vi "Get LV Timestamp Format String.vi"() -> (0 "timestamp string format":string="%Y-%m-%dT%H:%M:%S%3u%z")   [LabVIEW 2021, in "Logging.lvlib"]
doc: "Get the nearest-compliant format string for ISO 8601 that LabVIEW supports. After formatting a timestamp, use \"Fix LV Timestamp String.vi\" to make the formatted timestamp compliant with ISO 8601."
uses:
  Logging.lvlib
panel:
  out "Now":string
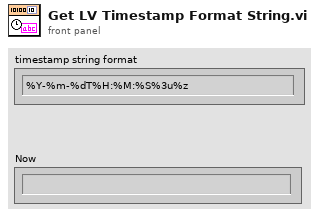
[diagram p1: front panel]
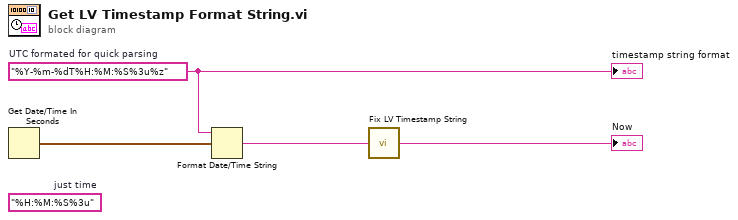
[diagram p0: block diagram]
diagram:
  (unwired) "%H:%M:%S%3u"  # just time
  w3 = "%Y-%m-%dT%H:%M:%S%3u%z"  # UTC formated for quick parsing
  n1 = Get Date/Time In Seconds() -> (seconds since 1Jan1904=w4:timestamp)
  n2 = Format Date/Time String(time format string (%c)=w3, seconds (now)=w4) -> (date/time string=w2:string)  [unwired: 1 in]
  n3 = call "Fix LV Timestamp String.vi"("LabVIEW format string"=w2) -> ("iso 8601 format string"=→"Now":string)
  "timestamp string format" <- w3
